vi "DDS Set RAM Profile.vi"(4 "Step Rate":u16, 5 "Profile (0)":u8, 6 "channel number (1)":u8=1 min=1 max=4 step=1, 7 "RAM mode":u8, 8 "error in (no error)":errorcluster, 9 "End Address":u16, 10 "Start Address":u16, 11 "DDS ref in":T1={"NI USB-8451 device reference"="", "DIO port"=0, "Serial Clock Rate [kHz]"=1000}) -> (0 "error out":errorcluster, 2 "Write Data":u8[](array[numeric]), 3 "DDS ref out":T1={"NI USB-8451 device reference"="", "DIO port"=0, "Serial Clock Rate [kHz]"=1000})   [LabVIEW 2013]
doc: "Program the RAM Profiles so they are ready to use the RAM settings."
uses:
  DDS_box_device_reference.ctl
  <vilib>/ni845x/ni845x.llb/ni845xControl.ctl
  AD9910 registers.ctl
  DDS RAM mode.ctl
  <vilib>/Utility/error.llb/DialogType.ctl
panel:
  out "mode":u8
  out "start add 2":u8
  out "start add 1":u8
  out "end add 2":u8
  out "end add 1":u8
  in  "No Dwell High":bool
  in  "Zero-crossing":bool
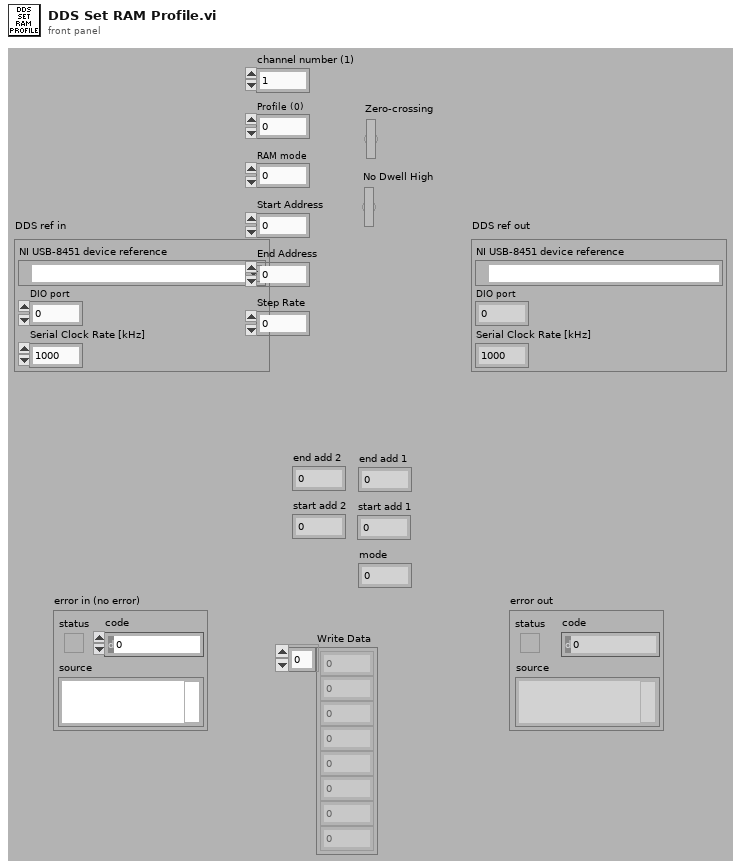
[diagram p1: front panel]
types:
  T1 = typedef "DDS_box_device_reference.ctl" = cluster{"NI USB-8451 device reference":T2, "DIO port":u8, "Serial Clock Rate [kHz]":u16}
  T2 = typedef "ni845xControl.ctl" = refnum<k21>
  T3 = typedef "DDS RAM mode.ctl" = enum16{"Direct Switch", "Ramp Up", "Bidirectional Ramp", "Continuous Bidirectional Ramp", "Continuous Recirculate", "Direct Switch 2", "Direct Switch 3", "Direct Switch 4"}
  T4 = typedef "AD9910 registers.ctl" = enum16{"CFR1", "CFR2", "CFR3", "Auxiliary DAC Control", "I/0 Update Rate", "Frequency Tuning Word", "Phase Offset Word", "Amplitude Scale Factor", "Multichip Sync", "Digital Ramp Limit", "Digital Ramp Step Size", "Digital Ramp Rate", "Single Tone Profile 0", "Single Tone Profile 1", "Single Tone Profile 2", "Single Tone Profile 3", "Single Tone Profile 4", "Single Tone Profile 5", "Single Tone Profile 6", "Single Tone Profile 7", "RAM Profile 0", "RAM Profile 1", "RAM Profile 2", "RAM Profile 3", "RAM Profile 4", "RAM Profile 5", "RAM Profile 6", "RAM Profile 7", "RAM"}
  T5 = typedef "DialogType.ctl" = u16
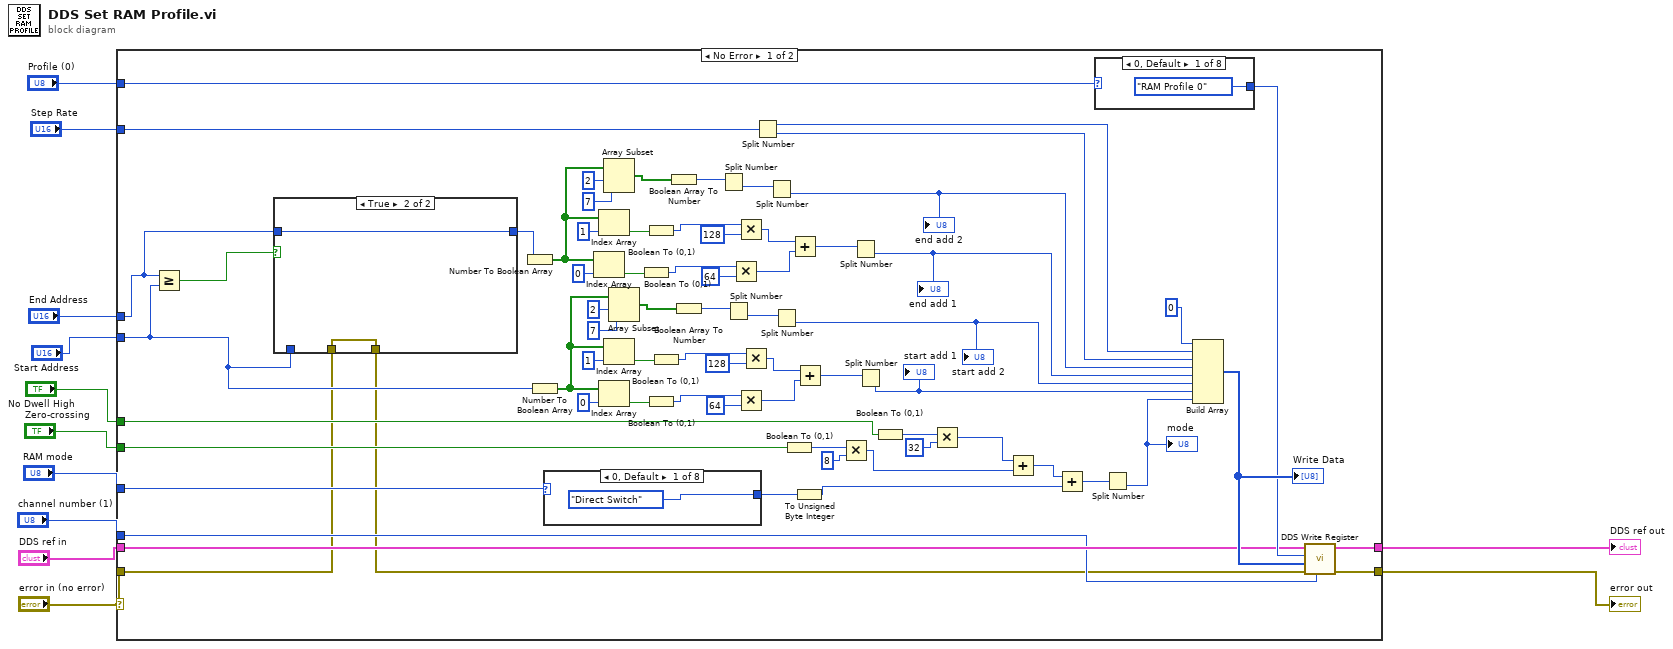
[diagram p0: block diagram]
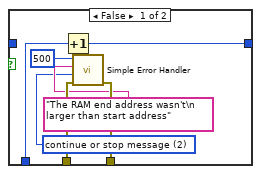
[diagram p2: hidden frame]
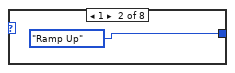
[diagram p3: hidden frame]
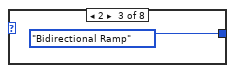
[diagram p4: hidden frame]
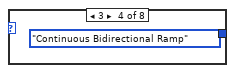
[diagram p5: hidden frame]
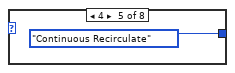
[diagram p6: hidden frame]
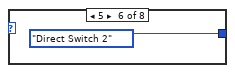
[diagram p7: hidden frame]
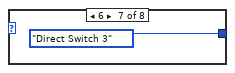
[diagram p8: hidden frame]
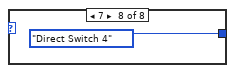
[diagram p9: hidden frame]
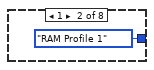
[diagram p10: hidden frame]
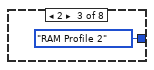
[diagram p11: hidden frame]
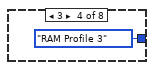
[diagram p12: hidden frame]
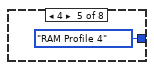
[diagram p13: hidden frame]
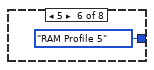
[diagram p14: hidden frame]
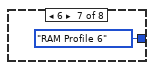
[diagram p15: hidden frame]
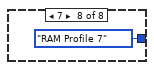
[diagram p16: hidden frame]
diagram:
  n1 = case shown="No Error" "error in (no error)" {
    tunnel: "error in (no error)" -> [w14 w108]
    tunnel: [w79 w108] -> w9
    tunnel: "Profile (0)" -> [w77 _]
    tunnel: "DDS ref in" -> [w76 w107]
    tunnel: [w78 w107] -> w8
    tunnel: "channel number (1)" -> [w75 _]
    tunnel: "RAM mode" -> [w74 _]
    tunnel: "Zero-crossing" -> [w61 _]
    tunnel: "No Dwell High" -> [w69 _]
    tunnel: "Start Address" -> [w15 _]
    tunnel: "End Address" -> [w17 _]
    tunnel: "Step Rate" -> [w21 _]
    frame No Error {
      n2 = Greater Or Equal?(x=w17, y=w15) -> (x >= y?=w18:bool)
      n3 = case shown="True" w18 {
        tunnel: w17 -> [_ w90]
        tunnel: [w88 w90] -> w16
        tunnel: w15 -> [w87 _]
        tunnel: w14 -> [w86 w89]
        tunnel: [w85 w89] -> w13
        frame False {
          w83 = T5 2 items=["no dialog", "OK message", "continue or stop message", "OK message + warnings", "continue/stop + warnings"] ("type of dialog (OK msg:1)")
          n4 = Increment(x=w87) -> (x+1=w88:u16)
          n5 = call <vilib>:"Simple Error Handler.vi"("error code (no error:0)"=500, "error source (\" \")"="The RAM end address wasn't\n larger than start address", "type of dialog (OK msg:1)"=w83, "error in (no error)"=w86) -> ("error out"=w85:errorcluster)  [unwired: 1 in, 4 out]
        }
        frame True {
        }
      }
      n6 = Number To Boolean Array(number=w16) -> (Boolean array=w30:bool[])
      n7 = Number To Boolean Array(number=w15) -> (Boolean array=w48:bool[])
      n8 = case shown="0, Default" w74 {
        tunnel: [DDS_RAM_mode."Direct Switch" ("RAM Mode") DDS_RAM_mode."Ramp Up" ("RAM Mode") DDS_RAM_mode."Bidirectional Ramp" ("RAM Mode") DDS_RAM_mode."Continuous Bidirectional Ramp" ("RAM Mode") DDS_RAM_mode."Continuous Recirculate" ("RAM Mode") DDS_RAM_mode."Direct Switch 2" ("RAM Mode") DDS_RAM_mode."Direct Switch 3" ("RAM Mode") DDS_RAM_mode."Direct Switch 4" ("RAM Mode")] -> w73
        frame 0, Default {
        }
        frame 1 {
        }
        frame 2 {
        }
        frame 3 {
        }
        frame 4 {
        }
        frame 5 {
        }
        frame 6 {
        }
        frame 7 {
        }
      }
      n9 = Index Array(array=w30, index=0) -> (element=w40:bool)
      n10 = Index Array(array=w30, index=1) -> (element=w36:bool)
      n11 = Index Array(array=w48, index=0) -> (element=w59:bool)
      n12 = Array Subset(array=w30, index=2, length=7) -> (w27:bool[])
      n13 = Index Array(array=w48, index=1) -> (element=w55:bool)
      n14 = Array Subset(array=w48, index=2, length=7) -> (w45:bool[])
      n15 = Boolean To (0,1)(Boolean=w40) -> (0, 1=w39:i16)
      n16 = Boolean To (0,1)(Boolean=w36) -> (0, 1=w35:i16)
      n17 = Boolean To (0,1)(Boolean=w59) -> (0, 1=w58:i16)
      n18 = Boolean To (0,1)(Boolean=w55) -> (0, 1=w54:i16)
      n19 = Boolean Array To Number(Boolean array=w27) -> (number=w26:u32)
      n20 = Boolean Array To Number(Boolean array=w45) -> (number=w44:u32)
      n21 = Split Number(x=w26) -> (lo(x)=w25:u16)  [unwired: 1 out]
      n22 = Split Number(x=w44) -> (lo(x)=w43:u16)  [unwired: 1 out]
      n23 = Multiply(x=w39, y=i16 64) -> (x*y=w32:i16)
      n24 = Multiply(x=w35, y=i16 128) -> (x*y=w33:i16)
      n25 = Multiply(x=w58, y=i16 64) -> (x*y=w51:i16)
      n26 = Multiply(x=w54, y=i16 128) -> (x*y=w52:i16)
      n27 = Split Number(x=w21) -> (hi(x)=w19:u8, lo(x)=w20:u8)
      n28 = Split Number(x=w25) -> (lo(x)=w23:u8)  [unwired: 1 out]
      "end add 2" <- w23
      n29 = Split Number(x=w43) -> (lo(x)=w42:u8)  [unwired: 1 out]
      "start add 2" <- w42
      n30 = Boolean To (0,1)(Boolean=w61) -> (0, 1=w71:i16)
      n31 = Add(x=w33, y=w32) -> (x+y=w31:i16)
      n32 = To Unsigned Byte Integer(number=w73) -> (unsigned 8bit integer=w65:u8)
      n33 = Add(x=w52, y=w51) -> (x+y=w50:i16)
      n34 = Multiply(x=w71, y=u8 8) -> (x*y=w66:i16)
      n35 = Split Number(x=w31) -> (lo(x)=w24:u8)  [unwired: 1 out]
      "end add 1" <- w24
      n36 = Split Number(x=w50) -> (lo(x)=w49:u8)  [unwired: 1 out]
      "start add 1" <- w49
      n37 = Boolean To (0,1)(Boolean=w69) -> (0, 1=w70:i16)
      n38 = Multiply(x=w70, y=u8 32) -> (x*y=w67:i16)
      n39 = Add(x=w67, y=w66) -> (x+y=w64:i16)
      n40 = Add(x=w64, y=w65) -> (x+y=w63:i16)
      n41 = case shown="0, Default" w77 {
        tunnel: [AD9910_registers."RAM Profile 0" ("Register") AD9910_registers."RAM Profile 1" ("Register") AD9910_registers."RAM Profile 2" ("Register") AD9910_registers."RAM Profile 3" ("Register") AD9910_registers."RAM Profile 4" ("Register") AD9910_registers."RAM Profile 5" ("Register") AD9910_registers."RAM Profile 6" ("Register") AD9910_registers."RAM Profile 7" ("Register")] -> w80
        frame 0, Default {
        }
        frame 1 {
        }
        frame 2 {
        }
        frame 3 {
        }
        frame 4 {
        }
        frame 5 {
        }
        frame 6 {
        }
        frame 7 {
        }
      }
      n42 = Split Number(x=w63) -> (lo(x)=w62:u8)  [unwired: 1 out]
      "mode" <- w62
      n43 = Build Array(u8 0 ("element"), w19, w20, w23, w24, w42, w49, w62) -> (w81:u8[])
      "Write Data" <- w81
      n44 = call "DDS Write Register.vi"("channel number (1)"=w75, "error in (no error)"=w13, "Write Data"=w81, "Register"=w80, "DDS ref in"=w76) -> ("error out"=w79:errorcluster, "DDS ref out"=w78:T1)  [unwired: 5 in]
    }
    frame Error {
    }
  }
  "error out" <- w9
  "DDS ref out" <- w8
